vi "toggle.vi"(1 "Btn In":bool) -> (0 "Toggle Out":bool)   [LabVIEW 2012]
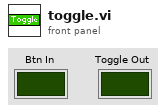
[diagram p1: front panel]
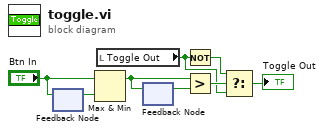
[diagram p0: block diagram]
diagram:
  n1 = feedback-in #1("Btn In") -> ()
  n2 = feedback #1() -> (w6:bool)  [unwired: 1 in]
  n3 = Max & Min(x="Btn In", y=w6) -> (max(x,y)=w5:bool)  [unwired: 1 out]
  n4 = local read "Toggle Out"() -> (w1:bool)
  n5 = feedback #2() -> (w8:bool)  [unwired: 1 in]
  n6 = feedback-in #2(w5) -> ()
  n7 = Not(x=w1) -> (.not. x?=w2:bool)
  n8 = Greater?(x=w5, y=w8) -> (0:w4:bool)
  n9 = Select(t=w2, s=w4, f=w1) -> (s? t:f=→"Toggle Out":bool)
